vi "merge fault lists.vi"(10 "rt faults":T3[](array[typedef]), 11 "faults in":T1[](array[typedef])) -> (3 "faults out":T1[](array[typedef]))   [LabVIEW 2013, in "main engine.lvlib"]
doc: "Adds a new set of faults to the main list, merging them one-by-one."
uses:
  main engine.lvlib
  worker library/rt fault.ctl
  <vilib>/NI/Tag Bus Module Framework/runtime/error classification.ctl
  <vilib>/NI/Tag Bus Module Framework/module configuration/TBM module configuration.lvclass
  <vilib>/NI/Module Execution Interface/Engine Runtime/Fault.ctl
  worker library/worker pool.lvlib
  <vilib>/NI/Tag Bus Module Framework/runtime/TBM module execution interface.lvclass
  <vilib>/NI/Module Execution Interface/Engine Runtime/Engine Runtime Interface.lvclass
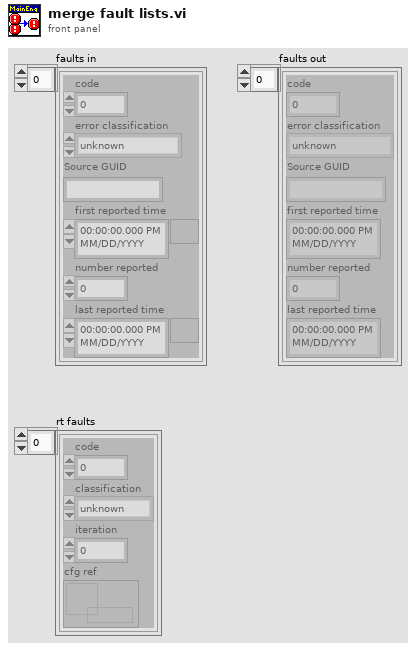
[diagram p1: front panel]
types:
  T1 = typedef "Engine Runtime Interface.lvclass/Fault.ctl" = cluster{"code":i32, "error classification":T2, "Source GUID":string, "first reported time":timestamp, "number reported":u32, "last reported time":timestamp}
  T2 = typedef "TBM module execution interface.lvclass/error classification.ctl" = enum16{"unknown", "none", "trivial", "recoverable", "critical"}
  T3 = typedef "worker pool.lvlib/rt fault.ctl" = cluster{"code":i32, "classification":T2, "iteration":u64, "cfg ref":refnum<data-value>}
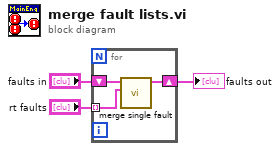
[diagram p0: block diagram]
diagram:
  n1 = for {
    shift-right: [w6] -> w2
    shift-left: "faults in" -> [w5]
    tunnel: "rt faults" -> [w4] mode=indexing
    n2 = call "merge single fault.vi"("new fault"=w4, "all faults in"=w5) -> ("all faults out"=w6:T1[])  [unwired: 9 in]
  }
  "faults out" <- w2
